vi "Global float Test VI.vi"() -> ()   [LabVIEW 2018]
panel:
  in  "New Value":dbl
  out "Boolean 4":bool
  out "Current value 4":dbl
  out "Boolean 3":bool
  out "Current value 3":dbl
  out "Boolean 2":bool
  out "Current value 2":dbl
  out "Boolean":bool
  out "Current value":dbl
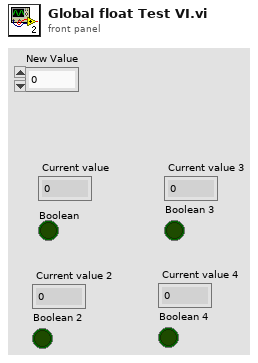
[diagram p1: front panel]
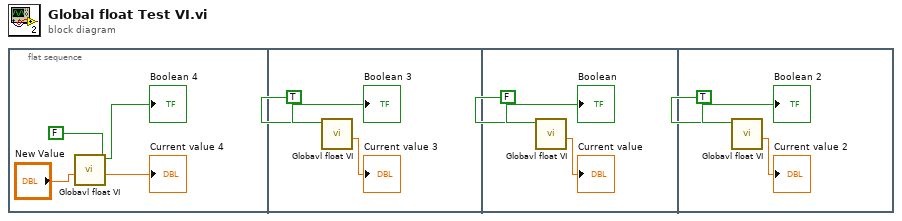
[diagram p0: block diagram]
diagram:
  n1 = flat-sequence {
    frame #0 {
      n2 = call "Globavl float VI.vi"("Set Value?"=FALSE, "New Value"="New Value") -> ("Current value"=→"Current value 4":dbl, "Boolean"=→"Boolean 4":bool)  [unwired: 8 in]
    }
    frame #1 {
      n3 = call "Globavl float VI.vi"("Set Value?"=TRUE) -> ("Current value"=→"Current value 3":dbl, "Boolean"=→"Boolean 3":bool)  [unwired: 9 in]
    }
    frame #2 {
      n4 = call "Globavl float VI.vi"("Set Value?"=FALSE) -> ("Current value"=→"Current value":dbl, "Boolean"=→"Boolean":bool)  [unwired: 9 in]
    }
    frame #3 {
      n5 = call "Globavl float VI.vi"("Set Value?"=TRUE) -> ("Current value"=→"Current value 2":dbl, "Boolean"=→"Boolean 2":bool)  [unwired: 9 in]
    }
  }
